vi "Universal_Ramping.vi"() -> ()   [LabVIEW 2015]
panel:
  out "Visa Command":string
  in  "milliseconds to wait":u32
  in  "VISA resource name":refnum<visa-resource-name>
  in  "Initial Voltage (V)":dbl caption="Initial Value"
  in  "Final Voltage (V)":dbl=0.1 caption="Final Value"
  in  "Voltage Step (V)":dbl=0.01 caption="Step Value"
  out "Increase/Decrease":string
  out "Ready":bool
  out "Actual Voltage (V)":dbl caption="Actual Value" step=0.1
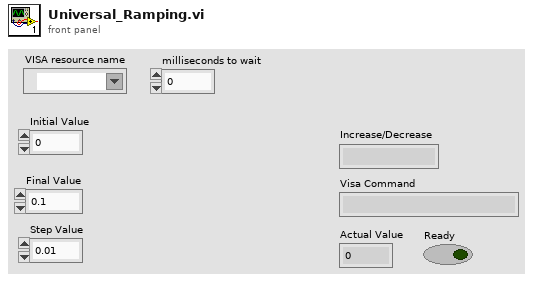
[diagram p1: front panel]
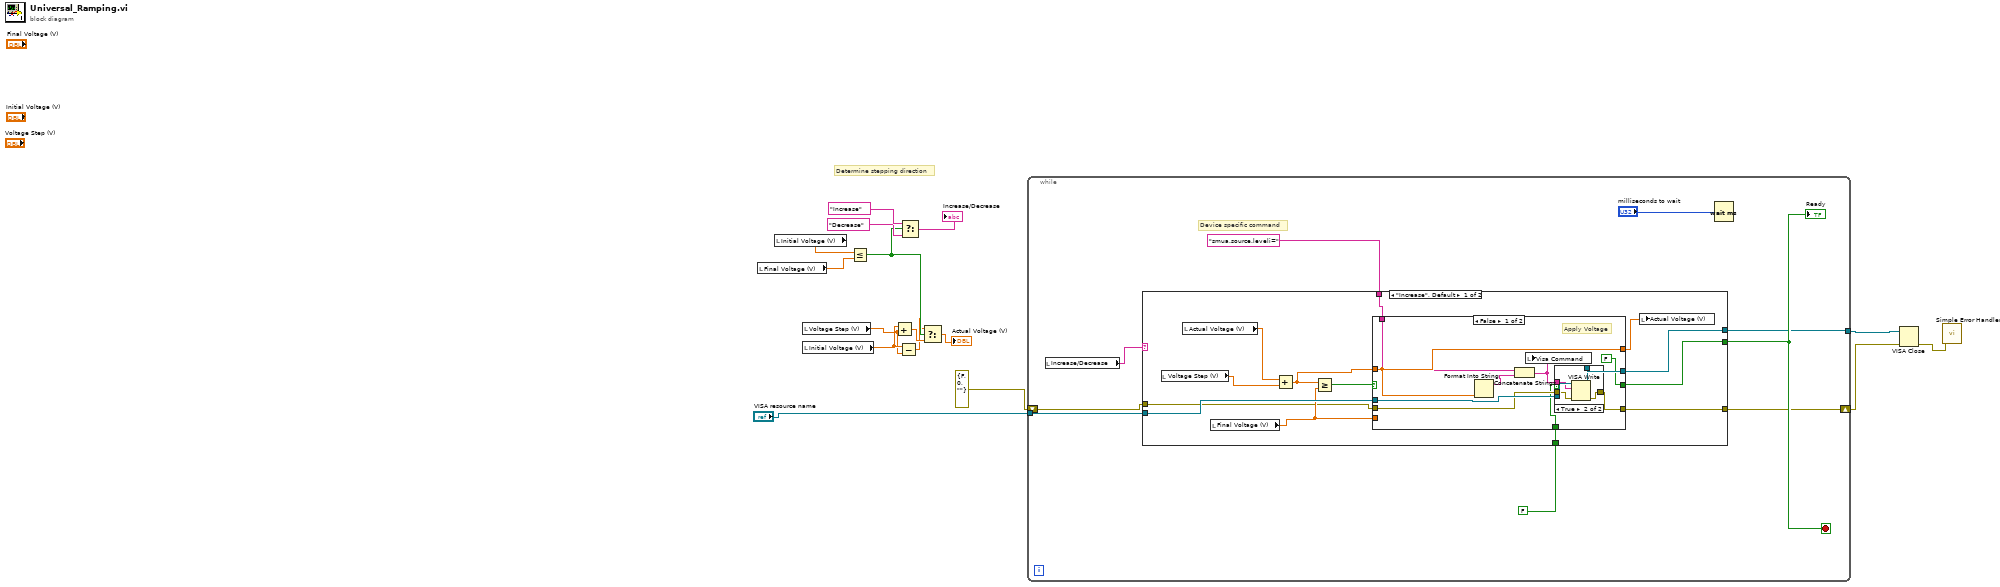
[diagram p0: block diagram]
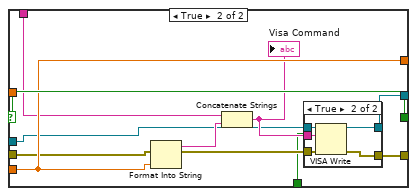
[diagram p3: hidden frame]
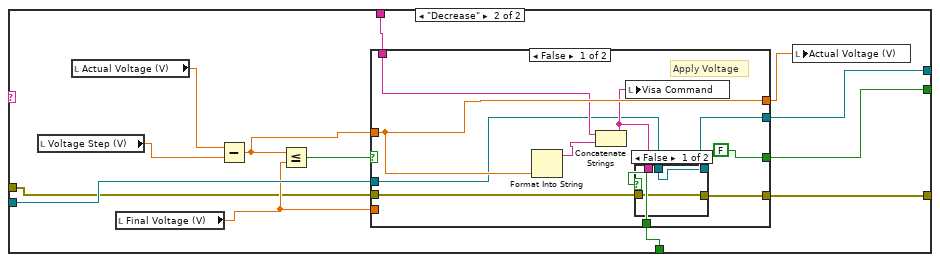
[diagram p5: hidden frame]
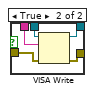
[diagram p6: hidden frame]
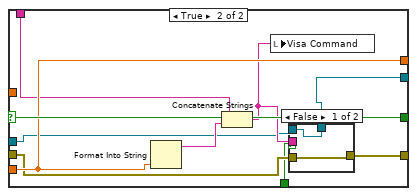
[diagram p7: hidden frame]
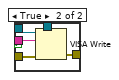
[diagram p8: hidden frame]
diagram:
  # "Determine stepping direction"
  n1 = local read "Final Voltage (V)"() -> (w14:dbl)
  n2 = local read "Initial Voltage (V)"() -> (w15:dbl)
  n3 = local read "Initial Voltage (V)"() -> (w8:dbl)
  n4 = local read "Voltage Step (V)"() -> (w7:dbl)
  n5 = Less Or Equal?(x=w15, y=w14) -> (x <= y?=w6:bool)
  n6 = Add(x=w8, y=w7) -> (x+y=w4:dbl)
  n7 = Subtract(x=w8, y=w7) -> (x-y=w3:dbl)
  n8 = Select(t="Increase", s=w6, f="Decrease") -> (s? t:f=→"Increase/Decrease":string)
  n9 = Select(t=w3, s=w6, f=w4) -> (s? t:f=→"Actual Voltage (V)":dbl)
  n10 = while {
    tunnel: "VISA resource name" -> [w24]
    tunnel: [w21] -> w10
    shift-right: [w18] -> w1
    shift-left: errorcluster {"status"=FALSE, "code"=0, "source"=""} ("error in (no error)") -> [w19]
    stop <- w25 stop-if-true
    # "Device specific command"
    n11 = local read "Increase/Decrease"() -> (w22:string)
    n12 = case shown="\"Increase\", Default" w22 {
      tunnel: [w35 w82] -> w25
      tunnel: w24 -> [w36 w83]
      tunnel: [w27 w77] -> w21
      tunnel: "smua.source.leveli=" ("write buffer") -> [w30 w76]
      tunnel: w19 -> [w29 w74]
      tunnel: [w28 w75] -> w18
      tunnel: FALSE -> [w26 w73]
      frame "Increase", Default {
        n13 = local read "Voltage Step (V)"() -> (w34:dbl)
        n14 = local read "Actual Voltage (V)"() -> (w33:dbl)
        n15 = local read "Final Voltage (V)"() -> (w31:dbl)
        n16 = Add(x=w33, y=w34) -> (x+y=w38:dbl)
        n17 = Greater Or Equal?(x=w38, y=w31) -> (x >= y?=w37:bool)
        n18 = case shown="False" w37 {
          selector: w37 -> [_ w65]
          tunnel: [FALSE w65] -> w35
          tunnel: w38 -> [w47 _]
          tunnel: w36 -> [w45 w58]
          tunnel: [w47 w63] -> w32
          tunnel: w31 -> [_ w63]
          tunnel: w30 -> [w46 w62]
          tunnel: w29 -> [w43 w60]
          tunnel: [w42 w59] -> w28
          tunnel: [w44 w57] -> w27
          tunnel: w26 -> [w40 w56]
          frame False {
            # "Apply Voltage"
            n19 = Format Into String(w47) -> (resulting string=w48:string)  [unwired: 3 in, 1 out]
            n20 = Concatenate Strings(w46, w48) -> (w41:string)
            n21 = local write "Visa Command"(w41) -> ()
            n22 = case shown="True" w40 {
              tunnel: w45 -> [w49 w55]
              tunnel: [w49 w54] -> w44
              tunnel: w43 -> [w50 w53]
              tunnel: [w50 w52] -> w42
              tunnel: w41 -> [_ w51]
              frame False {
              }
              frame True {
                n23 = VISA Write(VISA resource name=w55, write buffer=w51, error in (no error)=w53) -> (VISA resource name out=w54:refnum<visa-resource-name>, error out=w52:errorcluster)  [unwired: 1 out]
              }
            }
          }
          frame True {
            n24 = Format Into String(w63) -> (resulting string=w64:string)  [unwired: 3 in, 1 out]
            n25 = Concatenate Strings(w62, w64) -> (w61:string)
            "Visa Command" <- w61
            n26 = case shown="True" w56 {
              tunnel: w61 -> [_ w72]
              tunnel: w60 -> [w67 w71]
              tunnel: [w67 w70] -> w59
              tunnel: w58 -> [w66 w69]
              tunnel: [w66 w68] -> w57
              frame False {
              }
              frame True {
                n27 = VISA Write(VISA resource name=w69, write buffer=w72, error in (no error)=w71) -> (VISA resource name out=w68:refnum<visa-resource-name>, error out=w70:errorcluster)  [unwired: 1 out]
              }
            }
          }
        }
        n28 = local write "Actual Voltage (V)"(w32) -> ()
      }
      frame "Decrease" {
        n29 = local read "Voltage Step (V)"() -> (w81:dbl)
        n30 = local read "Actual Voltage (V)"() -> (w80:dbl)
        n31 = local read "Final Voltage (V)"() -> (w78:dbl)
        n32 = Subtract(x=w80, y=w81) -> (x-y=w85:dbl)
        n33 = Less Or Equal?(x=w85, y=w78) -> (x <= y?=w84:bool)
        n34 = case shown="False" w84 {
          selector: w84 -> [_ w112]
          tunnel: [FALSE w112] -> w82
          tunnel: w85 -> [w93 _]
          tunnel: w83 -> [w90 w107]
          tunnel: [w89 w106] -> w77
          tunnel: [w93 w110] -> w79
          tunnel: w78 -> [_ w110]
          tunnel: w76 -> [w92 w109]
          tunnel: [w88 w104] -> w75
          tunnel: w74 -> [w87 w105]
          tunnel: w73 -> [w86 w103]
          frame False {
            # "Apply Voltage"
            n35 = Format Into String(w93) -> (resulting string=w94:string)  [unwired: 3 in, 1 out]
            n36 = Concatenate Strings(w92, w94) -> (w91:string)
            n37 = local write "Visa Command"(w91) -> ()
            n38 = case shown="False" w86 {
              tunnel: w91 -> [_ w102]
              tunnel: w90 -> [w96 w101]
              tunnel: [w96 w100] -> w89
              tunnel: [w97 w99] -> w88
              tunnel: w87 -> [w97 w98]
              frame False {
              }
              frame True {
                n39 = VISA Write(VISA resource name=w101, write buffer=w102, error in (no error)=w98) -> (VISA resource name out=w100:refnum<visa-resource-name>, error out=w99:errorcluster)  [unwired: 1 out]
              }
            }
          }
          frame True {
            n40 = Format Into String(w110) -> (resulting string=w111:string)  [unwired: 3 in, 1 out]
            n41 = Concatenate Strings(w109, w111) -> (w108:string)
            n42 = local write "Visa Command"(w108) -> ()
            n43 = case shown="False" w103 {
              tunnel: w108 -> [_ w119]
              tunnel: w107 -> [w113 w118]
              tunnel: [w113 w117] -> w106
              tunnel: w105 -> [w114 w116]
              tunnel: [w114 w115] -> w104
              frame False {
              }
              frame True {
                n44 = VISA Write(VISA resource name=w118, write buffer=w119, error in (no error)=w116) -> (VISA resource name out=w117:refnum<visa-resource-name>, error out=w115:errorcluster)  [unwired: 1 out]
              }
            }
          }
        }
        n45 = local write "Actual Voltage (V)"(w79) -> ()
      }
    }
    "Ready" <- w25
    n46 = Wait (ms)(milliseconds to wait="milliseconds to wait") -> ()  [unwired: 1 out]
  }
  n47 = VISA Close(VISA resource name=w10, error in (no error)=w1) -> (error out=w9:errorcluster)
  n48 = call <vilib>:"Simple Error Handler.vi"("error in (no error)"=w9) -> ()  [unwired: 4 in, 5 out]
